vi "ENPH354_A2Q1.vi"() -> ()   [LabVIEW 2020]
panel:
  in  "stop":bool
  in  "Blink Frequency Control":i32(knob) scale=1.0..10.0
  out "Shift Register Method":bool
  out "Feedback Node Method":bool
  # "ENPH354 Assignment 2 Q1"
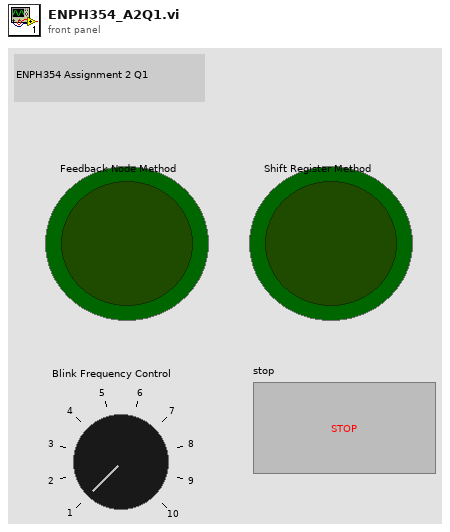
[diagram p1: front panel]
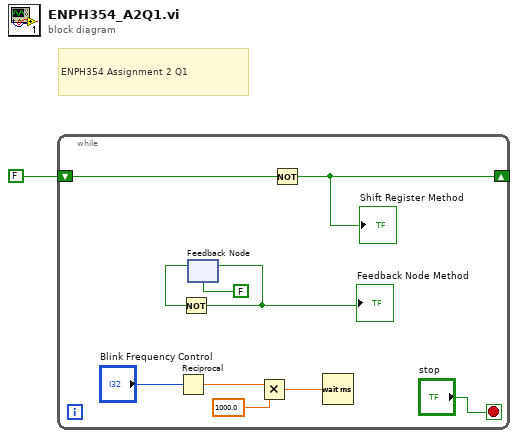
[diagram p0: block diagram]
diagram:
  # "ENPH354 Assignment 2 Q1"
  n1 = while {
    shift-right: [w2] -> _
    shift-left: FALSE -> [w10]
    stop <- "stop" stop-if-true
    n2 = Reciprocal(x="Blink Frequency Control") -> (1/x=w6:dbl)
    n3 = feedback #1(FALSE) -> (w5:bool)
    n4 = Not(x=w5) -> (.not. x?=w3:bool)
    "Feedback Node Method" <- w3
    n5 = feedback-in #1(w3) -> ()
    n6 = Multiply(x=w6, y=1000.0) -> (x*y=w9:dbl)
    n7 = Not(x=w10) -> (.not. x?=w2:bool)
    "Shift Register Method" <- w2
    n8 = Wait (ms)(milliseconds to wait=w9) -> ()  [unwired: 1 out]
  }
